vi "XY Message Loop.vi"(8 "error in (no error)":errorcluster, 10 "Data Notifiers":T1, 11 "Message Queues":T2) -> (0 "error out":errorcluster)   [LabVIEW 2013, in "XY.lvlib"]
uses:
  XY.lvlib
  support/Message Queue/All Message Queues.ctl
  support/Message Queue/Message Cluster.ctl
  support/Data Notifiers/All Data Notifiers.ctl
  Acquisition/APD Notifier Cluster.ctl
  Piezo/Piezo display.ctl
  XY Display.ctl
  Capacitive/Capacitive Signal Cluster.ctl
  XY Status.ctl
  Hardware Configuration.ctl
  support/Message Queue/Enqueue Message (Single).vi
  <vilib>/Utility/error.llb/Error Cluster From Error Code.vi
  <vilib>/ErrorRing/Error Ring.xnode
  support/Message Queue/Message Queue.lvlib
  Piezo/Piezo.lvlib
  Acquisition/Acquisition.lvlib
  support/Data Notifiers/Data Notifiers.lvlib
  Capacitive/Capacitive.lvlib
panel:
  in  "MG17Motor 2":refnum<k7>(container)
  in  "MG17Motor":refnum<k7>(container)
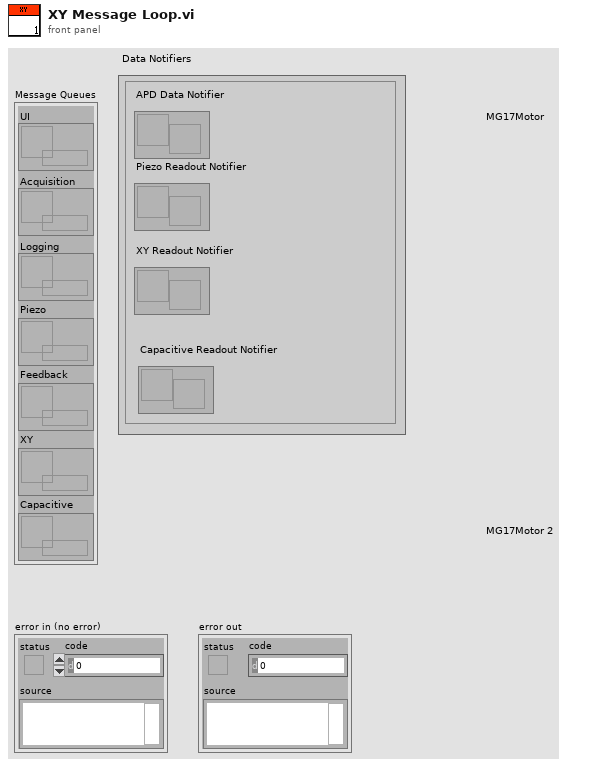
[diagram p1: front panel]
types:
  T1 = typedef "Data Notifiers.lvlib/All Data Notifiers.ctl" = cluster{"APD Data Notifier":refnum<notifier>, "Piezo Readout Notifier":refnum<notifier>, "XY Readout Notifier":refnum<notifier>, "Capacitive Readout Notifier":refnum<notifier>}
  T2 = typedef "Message Queue.lvlib/All Message Queues.ctl" = cluster{"UI":refnum<queue>, "Acquisition":refnum<queue>, "Logging":refnum<queue>, "Piezo":refnum<queue>, "Feedback":refnum<queue>, "XY":refnum<queue>, "Capacitive":refnum<queue>}
  T3 = typedef "XY.lvlib/Hardware Configuration.ctl" = cluster{"X refnum":refnum<k7>, "Y Refnum":refnum<k7>, "X Serial":i32, "Y Serial":i32, "X Setpoint":sgl, "Y Setpoint":sgl}
  T4 = typedef "XY.lvlib/XY Status.ctl" = enum16{"Idle", "Ready"}
  T5 = typedef "XY.lvlib/XY Display.ctl" = cluster{"X Position":sgl, "Y Position":sgl}
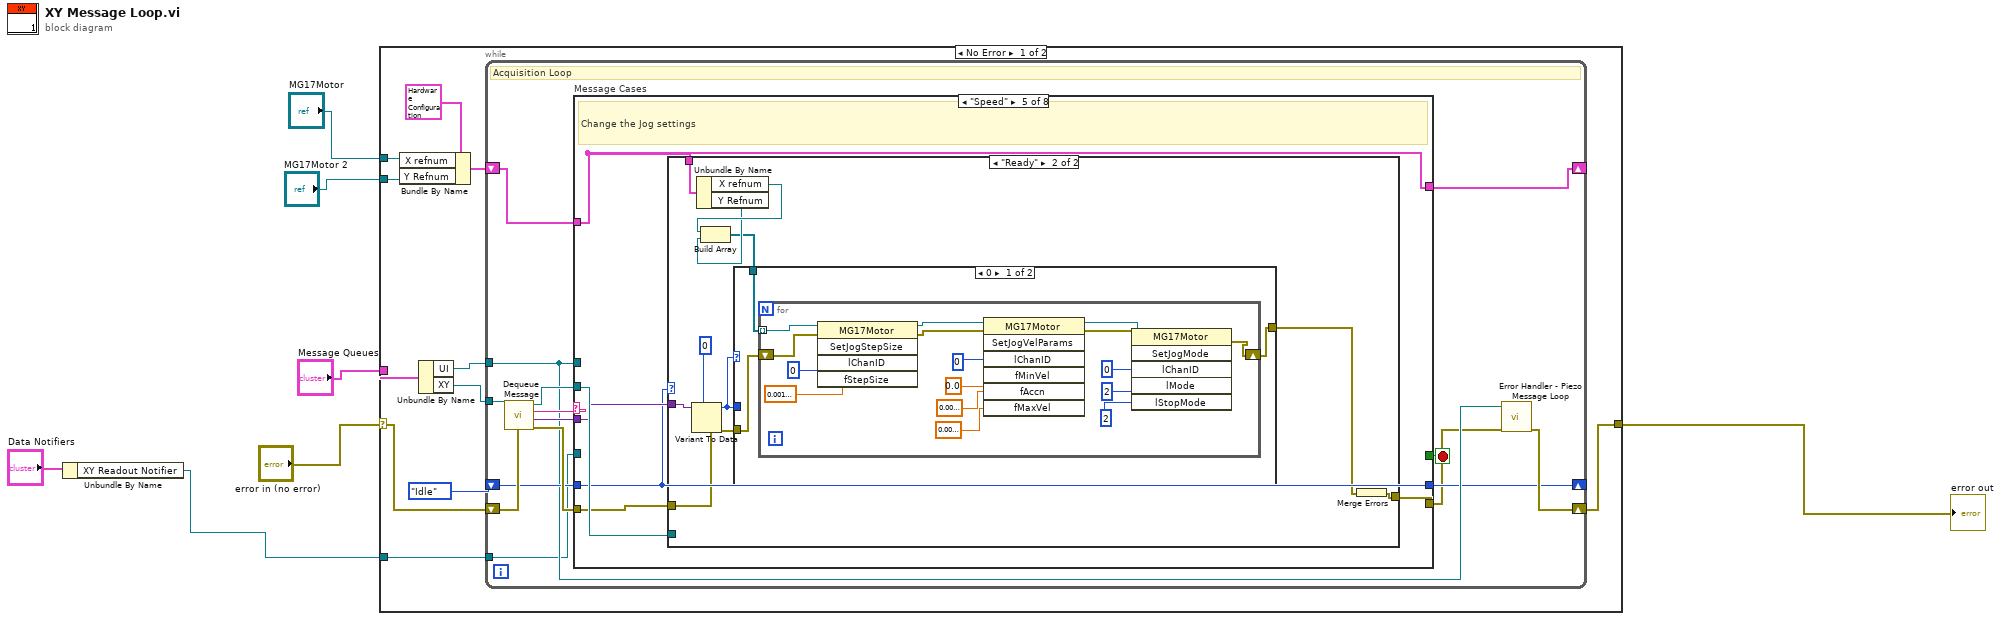
[diagram p0: block diagram]
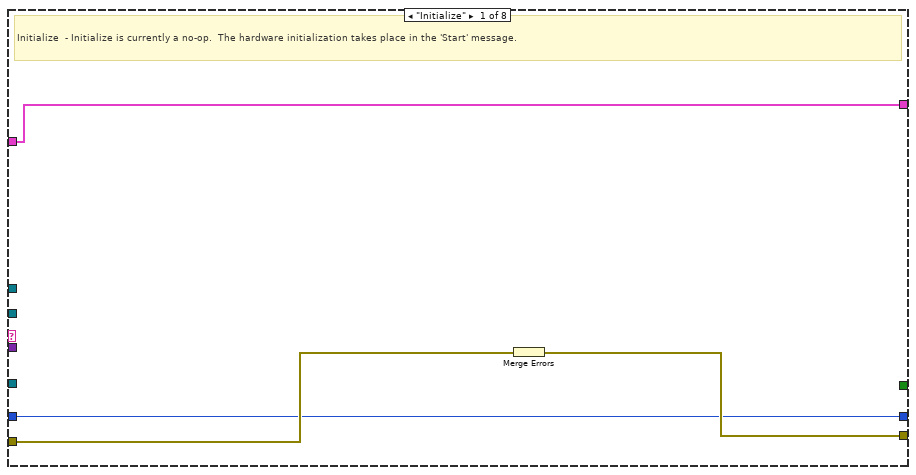
[diagram p2: hidden frame]
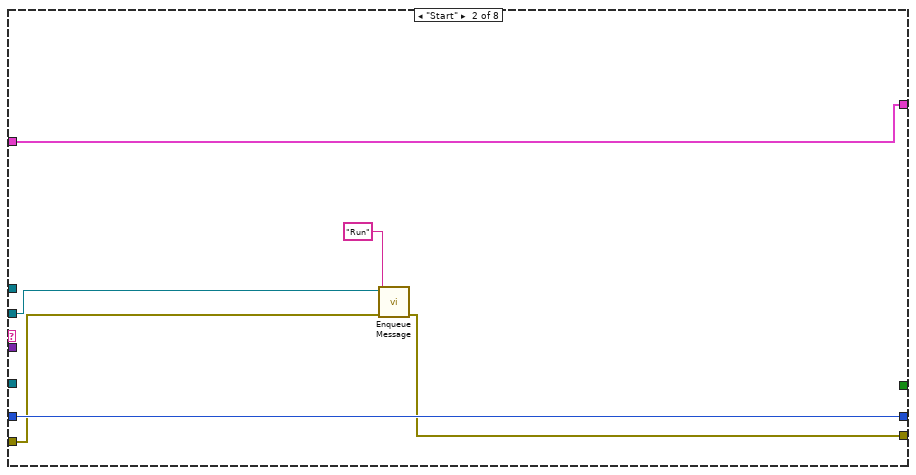
[diagram p3: hidden frame]
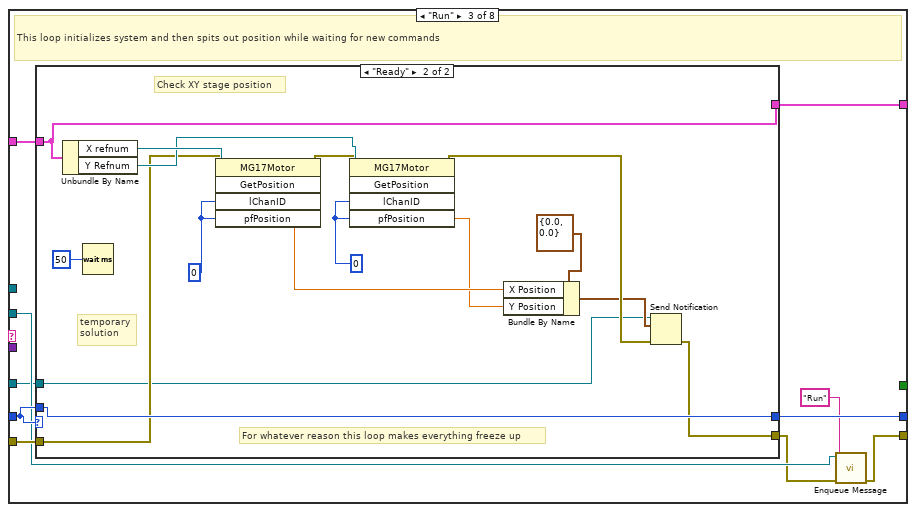
[diagram p4: hidden frame]
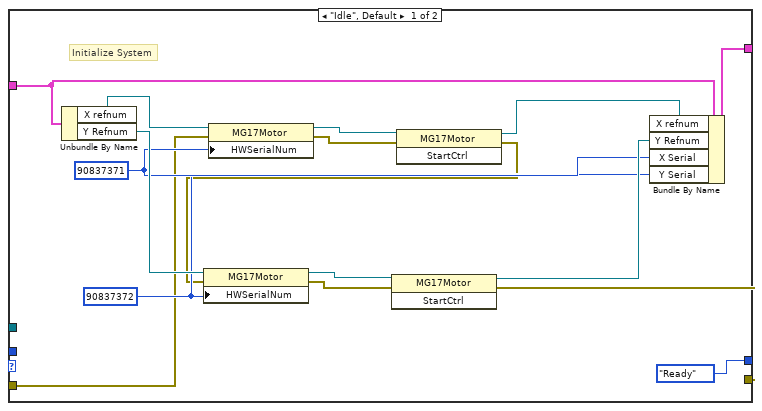
[diagram p5: hidden frame]
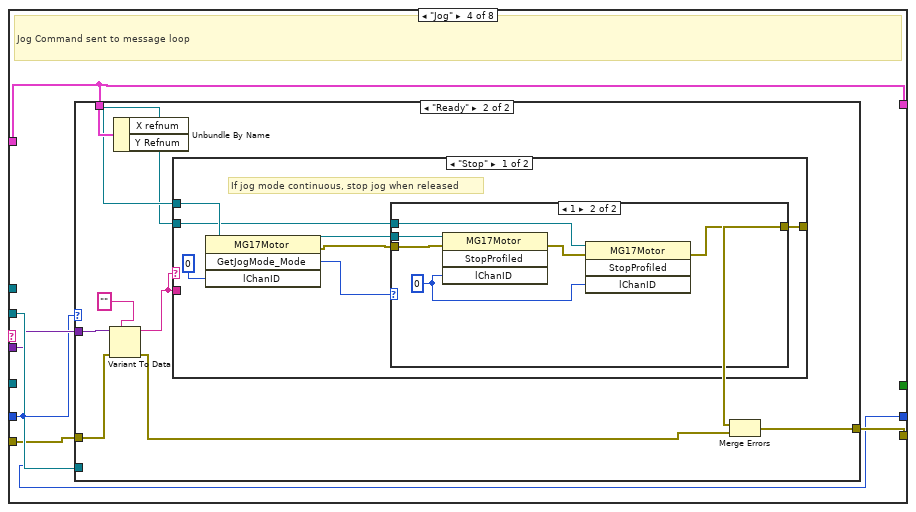
[diagram p6: hidden frame]
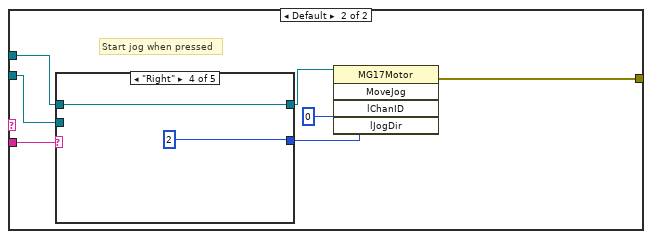
[diagram p9: hidden frame]
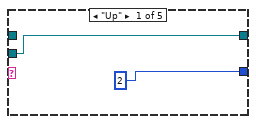
[diagram p10: hidden frame]
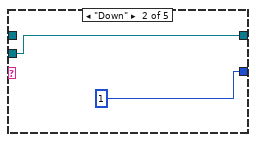
[diagram p11: hidden frame]
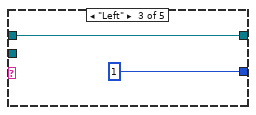
[diagram p12: hidden frame]
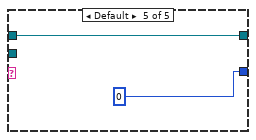
[diagram p13: hidden frame]
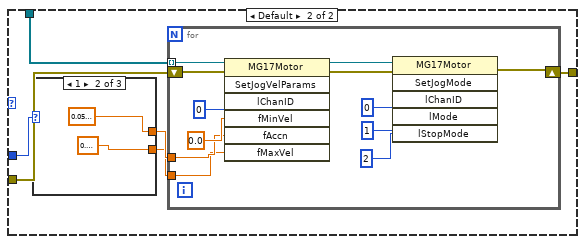
[diagram p15: hidden frame]
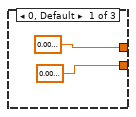
[diagram p16: hidden frame]
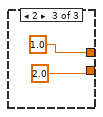
[diagram p17: hidden frame]
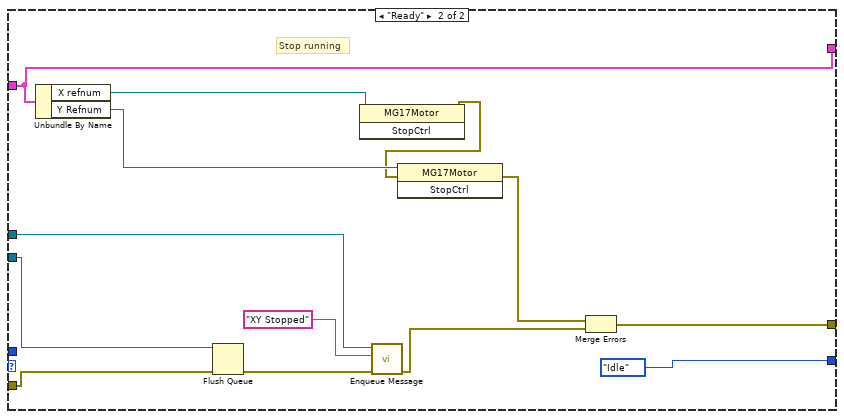
[diagram p19: hidden frame]
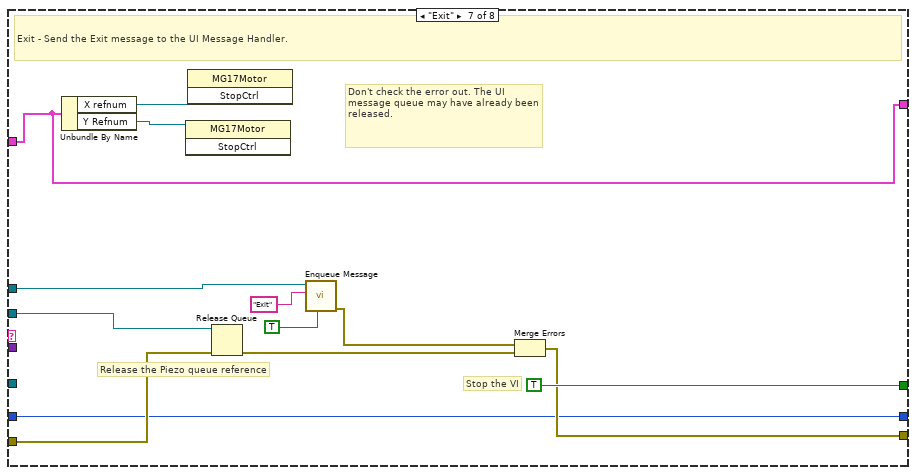
[diagram p20: hidden frame]
diagram:
  n1 = Unbundle By Name("Data Notifiers") -> ("XY Readout Notifier"=w1:refnum<notifier>)
  n2 = case shown="No Error" "error in (no error)" {
    selector: "error in (no error)" -> [w14 w243]
    tunnel: "Message Queues" -> [w18 _]
    tunnel: [w16 w243] -> w6
    tunnel: w1 -> [w13 _]
    tunnel: "MG17Motor" -> [w11 _]
    tunnel: "MG17Motor 2" -> [w10 _]
    frame No Error {
      n3 = Bundle By Name(cluster=T3 {"X refnum"=refnum, "Y Refnum"=refnum, "X Serial"=41848555, "Y Serial"=41848555, "X Setpoint"=0.0, "Y Setpoint"=0.0} ("XY Config"), "X refnum"=w11, "Y Refnum"=w10) -> (w8:T3)
      n4 = Unbundle By Name(w18) -> ("UI"=w15:refnum<queue>, "XY"=w17:refnum<queue>)
      n5 = while {
        tunnel: w17 -> [w27]
        shift-right: [w24] -> w16
        shift-left: w14 -> [w32]
        tunnel: w15 -> [w25]
        shift-right: [w23] -> _
        shift-left: XY_Status."Idle" ("XY Status") -> [w26]
        tunnel: w13 -> [w21]
        shift-right: [w19] -> _
        shift-left: w8 -> [w20]
        stop <- w33 stop-if-true
        # "Acquisition Loop"
        n6 = call "Dequeue Message.vi"("error in (no error)"=w32, "Message Queue"=w27) -> ("error out"=w31:errorcluster, "Message Data"=w29:variant, "Message"=w30:string, "dup Message Queue"=w28:refnum<queue>)  [unwired: 6 in]
        n7 = case "Message Cases" shown="\"Speed\"" w30 {
          selector: w30 -> [_ _ _ _ _ _ _ w235]
          tunnel: w28 -> [_ w40 w48 w91 w139 w197 w227 _]
          tunnel: w31 -> [w36 w39 w49 w88 w136 w196 w229 _]
          tunnel: [w37 w38 w45 w87 w135 w195 w230 w234] -> w22
          tunnel: [_ _ _ _ _ _ TRUE _] -> w33
          tunnel: w29 -> [_ _ _ w89 w137 _ _ _]
          tunnel: w25 -> [_ _ _ _ _ w198 w223 _]
          tunnel: w26 -> [w35 w41 w50 w86 w134 w199 w226 w233]
          tunnel: [w35 w41 w51 w86 w134 w200 w226 w233] -> w23
          tunnel: w21 -> [_ _ w44 _ _ _ _ _]
          tunnel: w20 -> [w34 w42 w53 w90 w138 w202 w219 w232]
          tunnel: [w34 w42 w52 w90 w138 w201 w219 w232] -> w19
          frame "Initialize" {
            # "Initialize  - Initialize is currently a no-op.  The hardware initialization takes place in the 'Start' message."
            n8 = Merge Errors(w36) -> (w37:errorcluster)
          }
          frame "Start" {
            n9 = call-poly "Enqueue Message.vi"("error in (no error)"=w39, "Message"="Run", "Message Queue"=w40) -> ("error out"=w38:errorcluster)  [unwired: 7 in, 1 out]
          }
          frame "Run" {
            # "This loop initializes system and then spits out position while waiting for new commands"
            n10 = case shown="\"Ready\"" w50 {
              tunnel: w53 -> [w61 w81]
              tunnel: [w60 w81] -> w52
              tunnel: [XY_Status."Ready" ("XY Status") w80] -> w51
              tunnel: w50 -> [_ w80]
              tunnel: w49 -> [w58 w79]
              tunnel: [w54 w70] -> w46
              tunnel: w44 -> [_ w71]
              frame "Idle", Default {
                w62 = 90837372 ("HWSerialNum")
                w63 = 90837371 ("HWSerialNum")
                # "Initialize System"
                n11 = Unbundle By Name(w61) -> ("X refnum"=w67:refnum<k7>, "Y Refnum"=w66:refnum<k7>)
                n12 = property class="MG17Motor"(reference=w67, error in=w58, "HWSerialNum"=w63) -> (reference out=w69:refnum<k7>, error out=w57:errorcluster)
                n13 = invoke class="MG17Motor" method="StartCtrl"(reference=w69, error in=w57) -> (reference out=w65:refnum<k7>, error out=w56:errorcluster)  [unwired: 1 in, 1 out]
                n14 = property class="MG17Motor"(reference=w66, error in=w56, "HWSerialNum"=w62) -> (reference out=w68:refnum<k7>, error out=w55:errorcluster)
                n15 = invoke class="MG17Motor" method="StartCtrl"(reference=w68, error in=w55) -> (reference out=w64:refnum<k7>, error out=w54:errorcluster)  [unwired: 1 in, 1 out]
                n16 = Bundle By Name(cluster=w61, "X refnum"=w65, "Y Refnum"=w64, "X Serial"=w63, "Y Serial"=w62) -> (w60:T3)
              }
              frame "Ready" {
                w84 = 0 ("lChanID")
                w85 = 0 ("lChanID")
                # "temporary\nsolution"
                # "For whatever reason this loop makes everything freeze up"
                # "Check XY stage position"
                n17 = Unbundle By Name(w81) -> ("X refnum"=w83:refnum<k7>, "Y Refnum"=w82:refnum<k7>)
                n18 = Wait (ms)(milliseconds to wait=u32 50) -> ()  [unwired: 1 out]
                n19 = invoke class="MG17Motor" method="GetPosition"(reference=w83, error in=w79, "lChanID"=w85, "pfPosition"=w85) -> (error out=w78:errorcluster, "pfPosition"=w75:sgl)  [unwired: 1 in, 3 out]
                n20 = invoke class="MG17Motor" method="GetPosition"(reference=w82, error in=w78, "lChanID"=w84, "pfPosition"=w84) -> (error out=w73:errorcluster, "pfPosition"=w74:sgl)  [unwired: 1 in, 3 out]
                n21 = Bundle By Name(cluster=T5 {"X Position"=0.0, "Y Position"=0.0} ("Cluster"), "X Position"=w75, "Y Position"=w74) -> (w72:T5)
                n22 = Send Notification(notification=w72, notifier=w71, error in (no error)=w73) -> (error out=w70:errorcluster)  [unwired: 1 out]
              }
            }
            n23 = call-poly "Enqueue Message.vi"("error in (no error)"=w46, "Message"="Run", "Message Queue"=w48) -> ("error out"=w45:errorcluster)  [unwired: 7 in, 1 out]
          }
          frame "Jog" {
            # "Jog Command sent to message loop"
            n24 = case shown="\"Ready\"" w86 {
              tunnel: w91 -> [_ _]
              tunnel: w90 -> [_ w102]
              tunnel: w89 -> [_ w101]
              tunnel: w88 -> [w92 w97]
              tunnel: [w92 w95] -> w87
              frame "Idle", Default {
              }
              frame "Ready" {
                n25 = Variant To Data(error in=w97, type="", Variant=w101) -> (data=w94:string, error out=w93:errorcluster)
                n26 = Unbundle By Name(w102) -> ("X refnum"=w99:refnum<k7>, "Y Refnum"=w98:refnum<k7>)
                n27 = case shown="\"Stop\"" w94 {
                  tunnel: w94 -> [_ w122]
                  tunnel: w99 -> [w109 w121]
                  tunnel: w98 -> [w104 w120]
                  tunnel: [w103 w117] -> w96
                  frame "Stop" {
                    # "If jog mode continuous, stop jog when released"
                    n28 = invoke class="MG17Motor" method="GetJogMode_Mode"(reference=w109, "lChanID"=0) -> (reference out=w106:refnum<k7>, error out=w105:errorcluster, "GetJogMode_Mode"=w107:i32)  [unwired: 2 in, 1 out]
                    n29 = case shown="1" w107 {
                      tunnel: w106 -> [_ w116]
                      tunnel: w105 -> [w110 w115]
                      tunnel: w104 -> [_ w112]
                      tunnel: [w110 w111] -> w103
                      frame 0, Default {
                      }
                      frame 1 {
                        w114 = 0 ("lChanID")
                        n30 = invoke class="MG17Motor" method="StopProfiled"(reference=w116, error in=w115, "lChanID"=w114) -> (error out=w113:errorcluster)  [unwired: 1 in, 3 out]
                        n31 = invoke class="MG17Motor" method="StopProfiled"(reference=w112, error in=w113, "lChanID"=w114) -> (error out=w111:errorcluster)  [unwired: 1 in, 3 out]
                      }
                    }
                  }
                  frame Default {
                    # "Start jog when pressed"
                    n32 = case shown="\"Right\"" w122 {
                      tunnel: w121 -> [_ _ w129 w131 w132]
                      tunnel: w120 -> [w125 w127 _ _ _]
                      tunnel: [w125 w127 w129 w131 w132] -> w119
                      tunnel: [2 ("lChanID") 1 ("lChanID") 1 ("lChanID") 2 ("lChanID") 0 ("lChanID")] -> w118
                      frame "Up" {
                      }
                      frame "Down" {
                      }
                      frame "Left" {
                      }
                      frame "Right" {
                      }
                      frame Default {
                      }
                    }
                    n33 = invoke class="MG17Motor" method="MoveJog"(reference=w119, "lChanID"=0, "lJogDir"=w118) -> (error out=w117:errorcluster)  [unwired: 2 in, 4 out]
                  }
                }
                n34 = Merge Errors(w96, w93) -> (w95:errorcluster)
              }
            }
          }
          frame "Speed" {
            # "Change the Jog settings"
            n35 = case shown="\"Ready\"" w134 {
              tunnel: w139 -> [_ _]
              tunnel: w138 -> [_ w151]
              tunnel: w137 -> [_ w150]
              tunnel: w136 -> [w140 w149]
              tunnel: [w140 w148] -> w135
              frame "Idle", Default {
              }
              frame "Ready" {
                n36 = Variant To Data(error in=w149, type=0 ("lChanID"), Variant=w150) -> (data=w141:i32, error out=w143:errorcluster)
                n37 = Unbundle By Name(w151) -> ("X refnum"=w146:refnum<k7>, "Y Refnum"=w145:refnum<k7>)
                n38 = Build Array(w146, w145) -> (w144:refnum<k7>[])
                n39 = case shown="0" w141 {
                  tunnel: w141 -> [_ w176]
                  tunnel: w144 -> [w154 w173]
                  tunnel: w143 -> [w153 w172]
                  tunnel: [w152 w171] -> w142
                  frame 0 {
                    n40 = for {
                      tunnel: w154 -> [w160] mode=indexing
                      shift-right: [w155] -> w152
                      shift-left: w153 -> [w156]
                      n41 = invoke class="MG17Motor" method="SetJogStepSize"(reference=w160, error in=w156, "lChanID"=0, "fStepSize"=sgl 0.001) -> (reference out=w159:refnum<k7>, error out=w161:errorcluster)  [unwired: 1 in, 3 out]
                      n42 = invoke class="MG17Motor" method="SetJogVelParams"(reference=w159, error in=w161, "lChanID"=0, "fMinVel"=sgl 0.0 ("pfMinVel"), "fAccn"=sgl 0.01, "fMaxVel"=sgl 0.01) -> (reference out=w165:refnum<k7>, error out=w164:errorcluster)  [unwired: 1 in, 5 out]
                      n43 = invoke class="MG17Motor" method="SetJogMode"(reference=w165, error in=w164, "lChanID"=0, "lMode"=2, "lStopMode"=2) -> (error out=w155:errorcluster)  [unwired: 1 in, 5 out]
                    }
                  }
                  frame Default {
                    n44 = case shown="1" w176 {
                      tunnel: [sgl 0.01 ("pfMinVel") sgl 0.05 ("pfMinVel") sgl 1.0 ("pfMinVel")] -> w175
                      tunnel: [sgl 0.01 ("pfMinVel") sgl 0.1 ("pfMinVel") sgl 2.0 ("pfMinVel")] -> w174
                      frame 0, Default {
                      }
                      frame 1 {
                      }
                      frame 2 {
                      }
                    }
                    n45 = for {
                      tunnel: w175 -> [w183]
                      tunnel: w174 -> [w182]
                      tunnel: w173 -> [w180] mode=indexing
                      shift-right: [w177] -> w171
                      shift-left: w172 -> [w179]
                      n46 = invoke class="MG17Motor" method="SetJogVelParams"(reference=w180, error in=w179, "lChanID"=0, "fMinVel"=sgl 0.0 ("pfMinVel"), "fAccn"=w183, "fMaxVel"=w182) -> (reference out=w181:refnum<k7>, error out=w178:errorcluster)  [unwired: 1 in, 5 out]
                      n47 = invoke class="MG17Motor" method="SetJogMode"(reference=w181, error in=w178, "lChanID"=0, "lMode"=1, "lStopMode"=2) -> (error out=w177:errorcluster)  [unwired: 1 in, 5 out]
                    }
                  }
                }
                n48 = Merge Errors(w142) -> (w148:errorcluster)
              }
            }
          }
          frame "Stop" {
            n49 = case shown="\"Idle\", Default" w199 {
              tunnel: w202 -> [w204 w218]
              tunnel: [w204 w218] -> w201
              tunnel: [w205 XY_Status."Idle" ("XY Status")] -> w200
              tunnel: w199 -> [w205 _]
              tunnel: w198 -> [_ w213]
              tunnel: w197 -> [_ w212]
              tunnel: w196 -> [w203 w209]
              tunnel: [w203 w206] -> w195
              frame "Idle", Default {
                # "Already Idle"
              }
              frame "Ready" {
                # "Stop running"
                n50 = Unbundle By Name(w218) -> ("X refnum"=w217:refnum<k7>, "Y Refnum"=w216:refnum<k7>)
                n51 = Flush Queue(queue=w212, error in (no error)=w209) -> (error out=w211:errorcluster)  [unwired: 2 out]
                n52 = invoke class="MG17Motor" method="StopCtrl"(reference=w217) -> (error out=w210:errorcluster)  [unwired: 2 in, 2 out]
                n53 = call-poly "Enqueue Message.vi"("error in (no error)"=w211, "Message"="XY Stopped", "Message Queue"=w213) -> ("error out"=w207:errorcluster)  [unwired: 7 in, 1 out]
                n54 = invoke class="MG17Motor" method="StopCtrl"(reference=w216, error in=w210) -> (error out=w208:errorcluster)  [unwired: 1 in, 2 out]
                n55 = Merge Errors(w208, w207) -> (w206:errorcluster)
              }
            }
          }
          frame "Exit" {
            # "Don't check the error out. The UI message queue may have already been released."
            # "Release the Piezo queue reference"
            # "Stop the VI"
            # "Exit - Send the Exit message to the UI Message Handler."
            n56 = Unbundle By Name(w219) -> ("X refnum"=w220:refnum<k7>, "Y Refnum"=w221:refnum<k7>)
            n57 = invoke class="MG17Motor" method="StopCtrl"(reference=w221) -> ()  [unwired: 2 in, 3 out]
            n58 = invoke class="MG17Motor" method="StopCtrl"(reference=w220) -> ()  [unwired: 2 in, 3 out]
            n59 = Release Queue(queue=w227, error in (no error)=w229) -> (error out=w228:errorcluster)  [unwired: 1 in, 2 out]
            n60 = call-poly "Enqueue Message.vi"("Priority Message? (F)"=TRUE, "Message"="Exit", "Message Queue"=w223) -> ("error out"=w222:errorcluster)  [unwired: 7 in, 1 out]
            n61 = Merge Errors(w222, w228) -> (w230:errorcluster)
          }
          frame Default {
            # "'Default' case only runs if there is a message that isn't defined in any of the other cases.  Output a programming error."
            n62 = xnode "Error Ring"("parameter 0"=w235) -> ("error out"=w234:errorcluster)
          }
        }
        n63 = call "Error Handler - Piezo Message Loop.vi"("error in (no error)"=w22, "Message Queue"=w25) -> ("dup error in"=w24:errorcluster)  [unwired: 8 in, 1 out]
      }
    }
    frame Error {
    }
  }
  "error out" <- w6
